vi "ReadFFLoop_thread.vi"(0 "blocktrigger":u8, 1 "btrig_ch":u8, 2 "ExtTrig":u8, 3 "cam_sel":u8, 5 "exptus":u32=20000) -> ()   [LabVIEW 2017]
uses:
  ESLSCDLL.dll
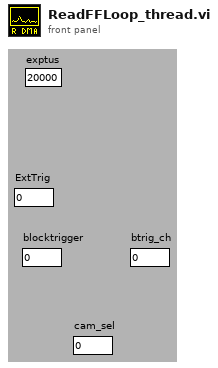
[diagram p1: front panel]
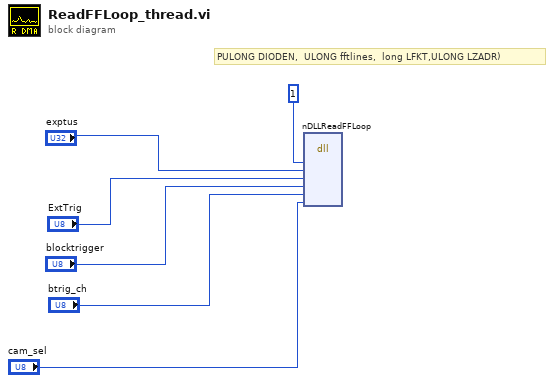
[diagram p0: block diagram]
diagram:
  # "PULONG DIODEN, \tULONG fftlines,  long LFKT,ULONG LZADR)"
  n1 = dll-call lib="C:/ENTW/PCIE/64bit/lv64/lv64_eventdriven/board.vis/ESLSCDLL.dll" fn="nDLLReadFFLoop" ("lwlscdll.dll:DLLReadFFLoop")("drv"=u32 1, "exptus"="exptus", "exttrig"="ExtTrig", "blocktrigger"="blocktrigger", "btrig_ch"="btrig_ch", "cam_sel"="cam_sel") -> ()  [unwired: 10 in, 2 out]
